vi "save to file v1.2.vi"(10 "Trial Number":dbl=1.0 min=1.0 max=5.0 step=1.0, 11 "Solar Cell Number":dbl=1.0 min=1.0 max=12.0 step=1.0 format="%0#2.2g") -> (2 "Path":string)   [LabVIEW 2014]
doc: "Writes simulated, timestamped data to a text file in ASCII format that can be read by spreadsheet applications.\nThe VI opens a new file or overwrites an existing file. It calls the subVI Acquire Data (Simulated).vi to generate a timestamped data array that contains (number of acquisition) sets of data, and its length is equal to (number of acquisitions)*(number of points/acquisition). The data is plotted on the graph one set at a time.\nThe VI also converts an array of data to a row of tab-separated columns, prepends to it the timestamp column, and terminates the row with the end of line character. Refer to the Read from Text File VI in this LLB and the spreadsheet examples for more file formats."
uses:
  <vilib>/Utility/error.llb/DialogType.ctl
  Instance           3 24Saved   save to file new .vi
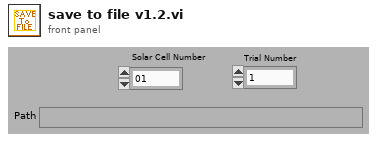
[diagram p1: front panel]
types:
  T1 = typedef "DialogType.ctl" = u16
  T2 = enum16{"open", "replace", "create", "open or create", "replace or create", "replace or create with confirmation"}
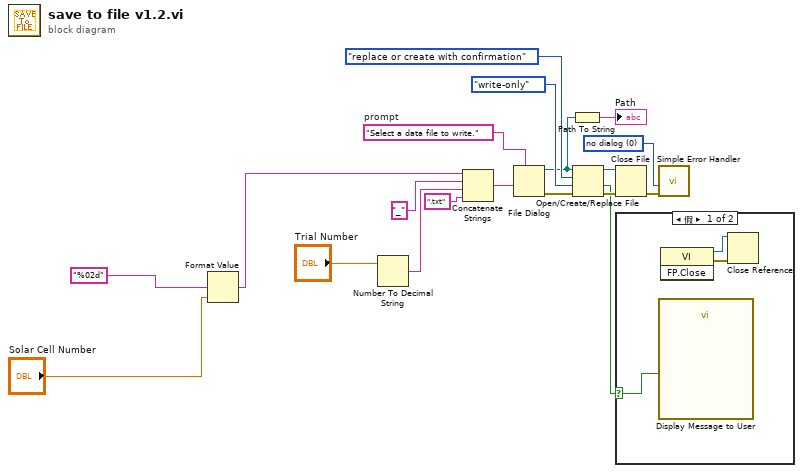
[diagram p0: block diagram]
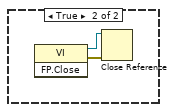
[diagram p2: hidden frame]
diagram:
  w10 = T1 0 items=["no dialog", "OK message", "continue or stop message", "OK message + warnings", "continue/stop + warnings"] ("type of dialog (OK msg:1)")
  w18 = "Select a data file to write."  # prompt
  n1 = Format Value(format string="%02d", value (0)="Solar Cell Number") -> (output string=w1:string)  [unwired: 1 out]
  n2 = Number To Decimal String(number="Trial Number") -> (decimal integer string=w8:string)  [unwired: 1 out]
  n3 = Concatenate Strings(w1, "_", w8, ".txt") -> (w5:string)
  n4 = File Dialog(7:w18, 9:w5) -> (0:w17:errorcluster, 3:w12:path)  [unwired: 1 in, 6 out]
  n5 = Path To String(path=w12) -> (string=→"Path":string)
  n6 = Open/Create/Replace File(file path (use dialog)=w12, error in=w17, operation (0:open)=T2."replace or create with confirmation", access (0:read/write)=enum16{"read/write", "read-only", "write-only"}."write-only") -> (refnum out=w13:refnum<file>, cancelled=w4:bool, error out=w14:errorcluster)  [unwired: 1 in, 1 out]
  n7 = Close File(refnum=w13, error in=w14) -> (error out=w19:errorcluster)  [unwired: 1 out]
  n8 = case shown="假" w4 {
    selector: w4 -> [w20 _]
    frame False {
      n9 = call "Display Message to User"("Enable"=w20) -> ()  [unwired: 2 in, 9 out]
      n10 = invoke class="VI" method="FP.Close"() -> (reference out=w21:refnum<vi>, error out=w22:errorcluster)  [unwired: 3 in, 1 out]
      n11 = Close Reference(reference=w21, error in (no error)=w22) -> ()  [unwired: 1 out]
    }
    frame True {
      n12 = invoke class="VI" method="FP.Close"() -> (reference out=w23:refnum<vi>, error out=w24:errorcluster)  [unwired: 3 in, 1 out]
      n13 = Close Reference(reference=w23, error in (no error)=w24) -> ()  [unwired: 1 out]
    }
  }
  n14 = call <vilib>:"Simple Error Handler.vi"("type of dialog (OK msg:1)"=w10, "error in (no error)"=w19) -> ()  [unwired: 8 out]
